vi "GOOP300_RemoveUnwantedChars.vi"(10 "StringIn":string) -> (2 "StringOut":string)   [LabVIEW 2020]
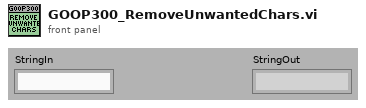
[diagram p1: front panel]
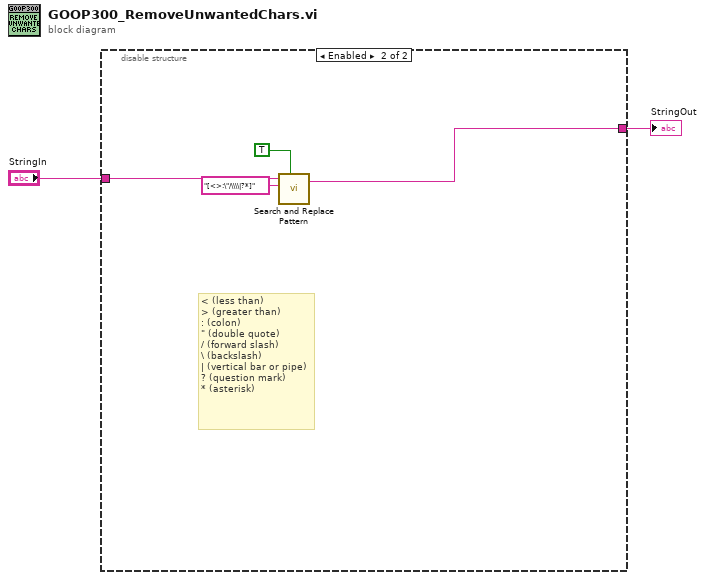
[diagram p0: block diagram]
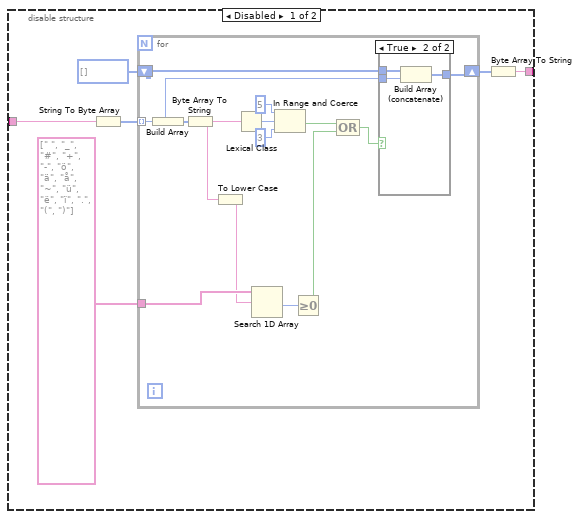
[diagram p2: hidden frame]
diagram:
  n1 = disable-structure shown="Enabled" {
    disable-tunnel: "StringIn" -> [w7 w30]
    disable-tunnel: [w4 w28] -> w1
    frame Disabled {
      n2 = String To Byte Array(string=w7) -> (unsigned byte array=w8:u8[])
      n3 = for {
        tunnel: w8 -> [w15] mode=indexing
        shift-right: [w16] -> w6
        shift-left: u8[] [] -> [w17]
        tunnel: string[] [" ", "_", "#", "+", "-", "ö", "ä", "å", "~", "ü", "ë", "ï", ".", "(", ")"] ("1D array") -> [w13]
        n4 = Build Array(w15) -> (w20:u8[])
        n5 = Byte Array To String(unsigned byte array=w20) -> (string=w11:string)
        n6 = To Lower Case(string=w11) -> (all lower case string=w10:string)
        n7 = Lexical Class(1:w11) -> (0:w18:i16)
        n8 = Search 1D Array(1D array=w13, element=w10) -> (index of element=w12:i32)  [unwired: 1 in]
        n9 = In Range and Coerce(upper limit=i16 5, x=w18, lower limit=i16 3) -> (In Range?=w19:bool)  [unwired: 1 out]
        n10 = Greater Or Equal To 0?(x=w12) -> (x >= 0?=w9:bool)
        n11 = Compound Arithmetic op=OR(w19, w9) -> (w14:bool)
        n12 = case shown="True" w14 {
          tunnel: w17 -> [w23 w26]
          tunnel: [w23 w25] -> w16
          tunnel: w15 -> [_ w24]
          frame False {
          }
          frame True {
            n13 = Build Array (concatenate)(w26, w24) -> (w25:u8[])
          }
        }
      }
      n14 = Byte Array To String(unsigned byte array=w6) -> (string=w4:string)
    }
    frame Enabled {
      # "< (less than)\n> (greater than)\n: (colon)\n\" (double quote)\n/ (forward slash)\n\\ (backslash)\n| (vertical bar or pipe)\n? (question mark)\n* (asterisk)"
      n15 = call <vilib>:"Search and Replace Pattern.vi"("string"=w30, "regular expression (\"\")"="[<>:\"/\\\\|?*]" ("regular expression (\"\")"), "replace all? (F)"=TRUE) -> ("result string"=w28:string)  [unwired: 2 in, 1 out]
    }
  }
  "StringOut" <- w1
